vi "ReadCANStatus.vi"(8 "error in (no error)":errorcluster caption="错误输入（无错误）", 9 "CANInd":u32, 10 "DeciceInd":u32, 11 "DeviceType":u32) -> (0 "error out":errorcluster caption="错误输出", 2 "VCI_CAN_STATUS":T1, 3 "Valid":bool)   [LabVIEW 2011]
uses:
  data/ControlCAN.dll
panel:
  # "typedef struct _VCI_CAN_STATUS{\n\tUCHAR\tErrInterrupt;\n\tUCHAR\tregMode;\n\tUCHAR\tregStatus;\n\tUCHAR\tregALCapture;\n\tUCHAR\tregECCapture; \n\tUCHAR\tregEWLimit;\n\tUCHAR\tregRECounter; \n\tUCHAR\tregTECounter;\n\tDWORD\tReserved;\n}VCI_CAN_STATUS,*PVCI_CAN_STATUS;"
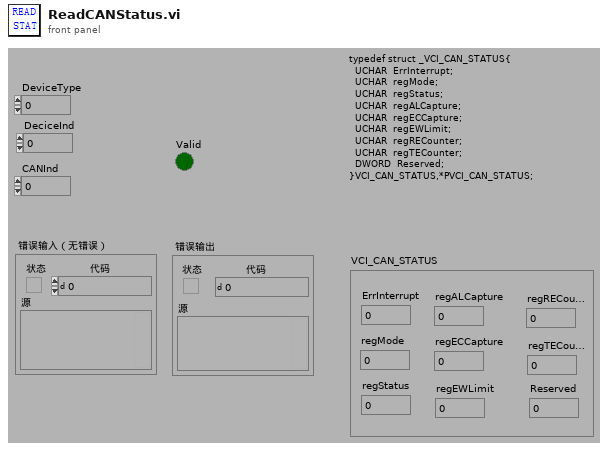
[diagram p1: front panel]
types:
  T1 = cluster{"ErrInterrupt":u8, "regMode":u8, "regStatus":u8, "regALCapture":u8, "regECCapture":u8, "regEWLimit":u8, "regRECounter":u8, "regTECounter":u8, "Reserved":u32}
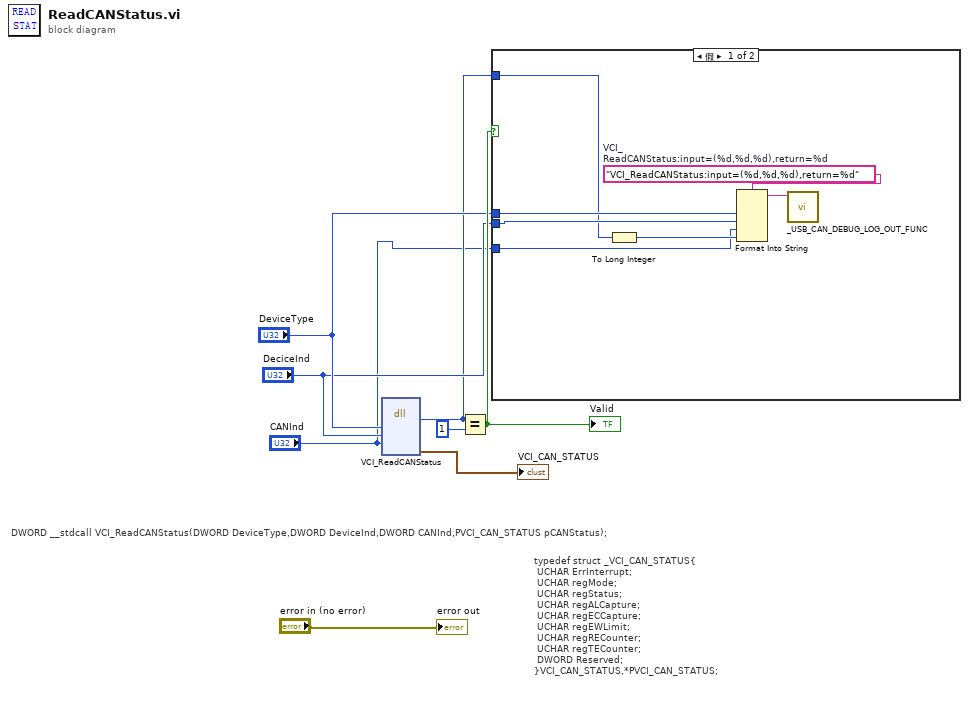
[diagram p0: block diagram]
diagram:
  # "typedef struct _VCI_CAN_STATUS{\n\tUCHAR\tErrInterrupt;\n\tUCHAR\tregMode;\n\tUCHAR\tregStatus;\n\tUCHAR\tregALCapture;\n\tUCHAR\tregECCapture; \n\tUCHAR\tregEWLimit;\n\tUCHAR\tregRECounter; \n\tUCHAR\tregTECounter;\n\tDWORD\tReserved;\n}VCI_CAN_STATUS,*PVCI_CAN_STATUS;"
  # "DWORD __stdcall VCI_ReadCANStatus(DWORD DeviceType,DWORD DeviceInd,DWORD CANInd,PVCI_CAN_STATUS pCANStatus);"
  n1 = dll-call lib="PTH1Mabs ZHost_E工作TnewcodeUSB CAN Tool1.97dataControlCAN.dll" fn="VCI_ReadCANStatus" label="VCI_StartCAN"("DeviceType"="DeviceType", "DeciceInd"="DeciceInd", "CANInd"="CANInd") -> ("返回类型"=w2:u32, "VCI_CAN_STATUS"=→"VCI_CAN_STATUS":T1)  [unwired: 7 in, 2 out]
  n2 = Equal?(x=w2, y=u32 1) -> (x = y?=w5:bool)
  "Valid" <- w5
  n3 = case shown="假" w5 {
    tunnel: "DeviceType" -> [w14 _]
    tunnel: "DeciceInd" -> [w13 _]
    tunnel: w2 -> [w12 _]
    tunnel: "CANInd" -> [w9 _]
    frame False {
      w11 = "VCI_ReadCANStatus:input=(%d,%d,%d),return=%d"  # VCI_ReadCANStatus:input=(%d,%d,%d),return=%d
      n4 = To Long Integer(number=w12) -> (32bit integer=w10:i32)
      n5 = Format Into String(format string=w11, w14, w13, w9, w10) -> (resulting string=w15:string)  [unwired: 2 in, 1 out]
      n6 = call "_USB_CAN_DEBUG_LOG_OUT_FUNC.vi"("Info"=w15) -> ()  [unwired: 11 in]
    }
    frame True {
    }
  }
  "error out" <- "error in (no error)"
